vi "Generate Timing Table.vi"(8 "error in (no error)":errorcluster, 11 "Performance Analyzer In":T1) -> (0 "error out":errorcluster, 2 "Timing List":string[](array[string]), 3 "Performance Analyzer Out":T1)   [LabVIEW 2020]
uses:
  Data Cluster.ctl
  Helper Classes/Test Finder/Test Finder.lvclass
  7fd359c0-f9a4-44c8-ab9e-fb113b9514a8.vi
  <vilib>/Array/Sort 2D Array - Pop Stack.vi
  <vilib>/Array/Sort 2D Array - Push Stack.vi
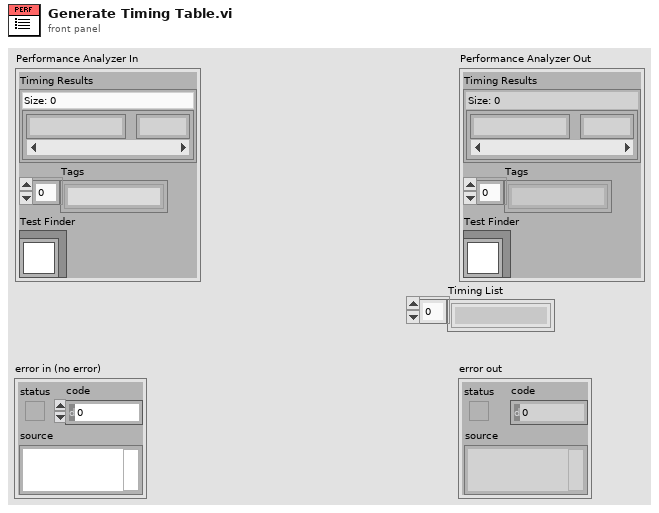
[diagram p1: front panel]
types:
  T1 = typedef "Data Cluster.ctl" = cluster{"Timing Results":map{string, dbl}, "Tags":string[], "Test Finder":refnum<class "Test Finder.lvclass">}
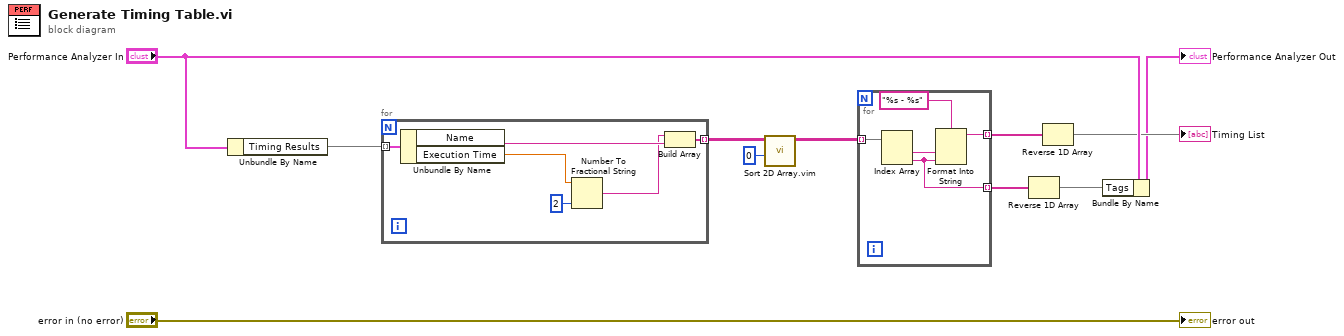
[diagram p0: block diagram]
diagram:
  n1 = Unbundle By Name("Performance Analyzer In") -> ("Timing Results"=w9:map{string, dbl})
  n2 = for {
    tunnel: w9 -> [w17] mode=indexing
    tunnel: [w13] -> w8 mode=indexing
    n3 = Unbundle By Name(w17) -> ("Name"=w16:string, "Execution Time"=w12:dbl)
    n4 = Number To Fractional String(number=w12, precision (6)=i16 2) -> (F-format string=w14:string)  [unwired: 2 in]
    n5 = Build Array(w14, w16) -> (w13:string[])
  }
  n6 = call "Sort 2D Array.vim"("index"=0, "2D array"=w8) -> ("sorted 2D array"=w6:string[][])  [unwired: 8 in, 1 out]
  n7 = for {
    tunnel: w6 -> [w22] mode=indexing
    tunnel: [w19] -> w5 mode=indexing
    tunnel: [w18] -> w3 mode=indexing
    n8 = Index Array(array=w22) -> (element #1=w20:string, element #2=w18:string)  [unwired: 2 in]
    n9 = Format Into String(format string="%s - %s", w20, w18) -> (resulting string=w19:string)  [unwired: 2 in, 1 out]
  }
  n10 = Reverse 1D Array(array=w3) -> (reversed array=w1:string[])
  n11 = Reverse 1D Array(array=w5) -> (reversed array=→"Timing List":string[])
  n12 = Bundle By Name(cluster="Performance Analyzer In", "Tags"=w1) -> (→"Performance Analyzer Out":T1)
  "error out" <- "error in (no error)"
